vi "sequential on_off - v2.vi"() -> ()   [LabVIEW 2018]
doc: "Manually blink and LED attached to a digital output channel of a LINX device by clicking and LED control in LabVIEW."
uses:
  <vilib>/MakerHub/LINX/Public/Peripherals/Digital/Digital Write 1 Chan.vi
  <vilib>/MakerHub/LINX/Public/Peripherals/Digital/Digital Write N Chans.vi
  <vilib>/MakerHub/LINX/Private/Local IO/LinxDigitalWrite.vi
  <vilib>/MakerHub/LINX/Public/Utilities/Check Channel.vi
  <vilib>/MakerHub/LINX/Public/Utilities/Open Serial.vi
  <vilib>/MakerHub/LINX/Private/Utilties/Generate Error.vi
  <vilib>/MakerHub/LINX/LMH-LINX.lvlib
panel:
  in  "Chnl_1":bool
  in  "Chnl_2":bool
  in  "Chnl_4":bool
  in  "Chnl_3":bool
  in  "Delay (ms)":dbl
  in  "Mode Selection":enum32{"Manual Control", "Sequential Control"}(radio)
  out "ch_4":bool
  out "ch_3":bool
  out "ch_2":bool
  out "ch_1":bool
  in  "Reset valves":bool
  out "id_8":bool
  out "id_7":bool
  out "id_6":bool
  out "id_5":bool
  out "id_4":bool
  out "id_3":bool
  out "id_2":bool
  out "id_1":bool
  in  "stop":bool
  in  "Valve 8":bool
  in  "Valve 7":bool
  in  "Valve 6":bool
  in  "Valve 5":bool
  in  "Valve 4":bool
  in  "Valve 3":bool
  in  "Valve 2":bool
  in  "Valve_1":bool
  in  "Serial Port":refnum<visa-resource-name>
  # "Manual Control:"
  # "LINX Device Settings"
  # "Sequential Control:"
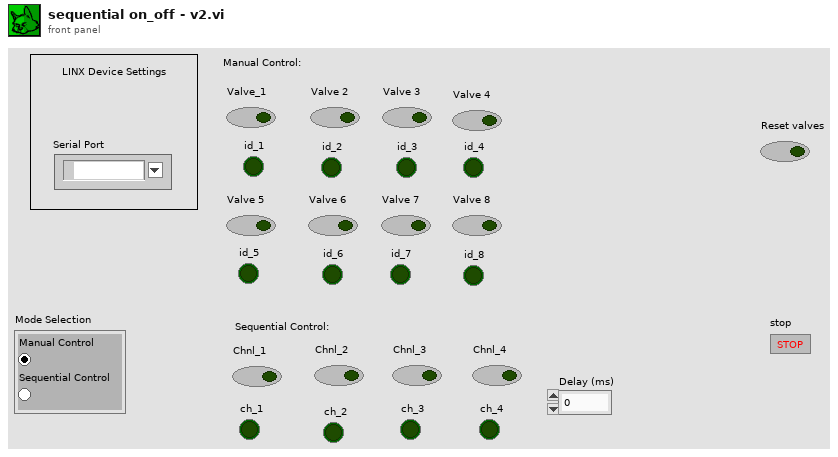
[diagram p1: front panel]
types:
  T1 = typedef "LMH-LINX.lvlib/LINX Ref.ctl" = cluster{"IO":T2, "Interface":T3, "LINX Device Config":T4}
  T2 = typedef "LMH-LINX.lvlib/Platform.ctl" = enum16{"Remote", "Local"}
  T3 = typedef "LMH-LINX.lvlib/Interface.ctl" = enum16{"Serial", "TCP"}
  T4 = typedef "LMH-LINX.lvlib/Device.lvlib/LINX Device Config.ctl" = cluster{"Interface":T3, "COM Port":refnum<visa-resource-name>, "TCP Configuration":T5, "Device Family":u8, "Device ID":u8, "Device Name":string, "TCP Ref":refnum<k5>, "Channels":T6}
  T5 = typedef "LMH-LINX.lvlib/Device.lvlib/TCP Config.ctl" = cluster{"IP Address":string, "Port":u16}
  T6 = typedef "LMH-LINX.lvlib/Channels.ctl" = cluster{"DI":u8[], "DO":u8[], "AI":u8[], "AO":u8[], "PWM":u8[], "QE":u8[], "UART":u8[], "I2C 2":u8[], "SPI":u8[], "CAN":u8[], "Servo":u8[], "AI Ref (V)":dbl, "AI Resolution (Bits)":u8, "AO Ref (V)":dbl, "AO Resolution (Bits)":u8}
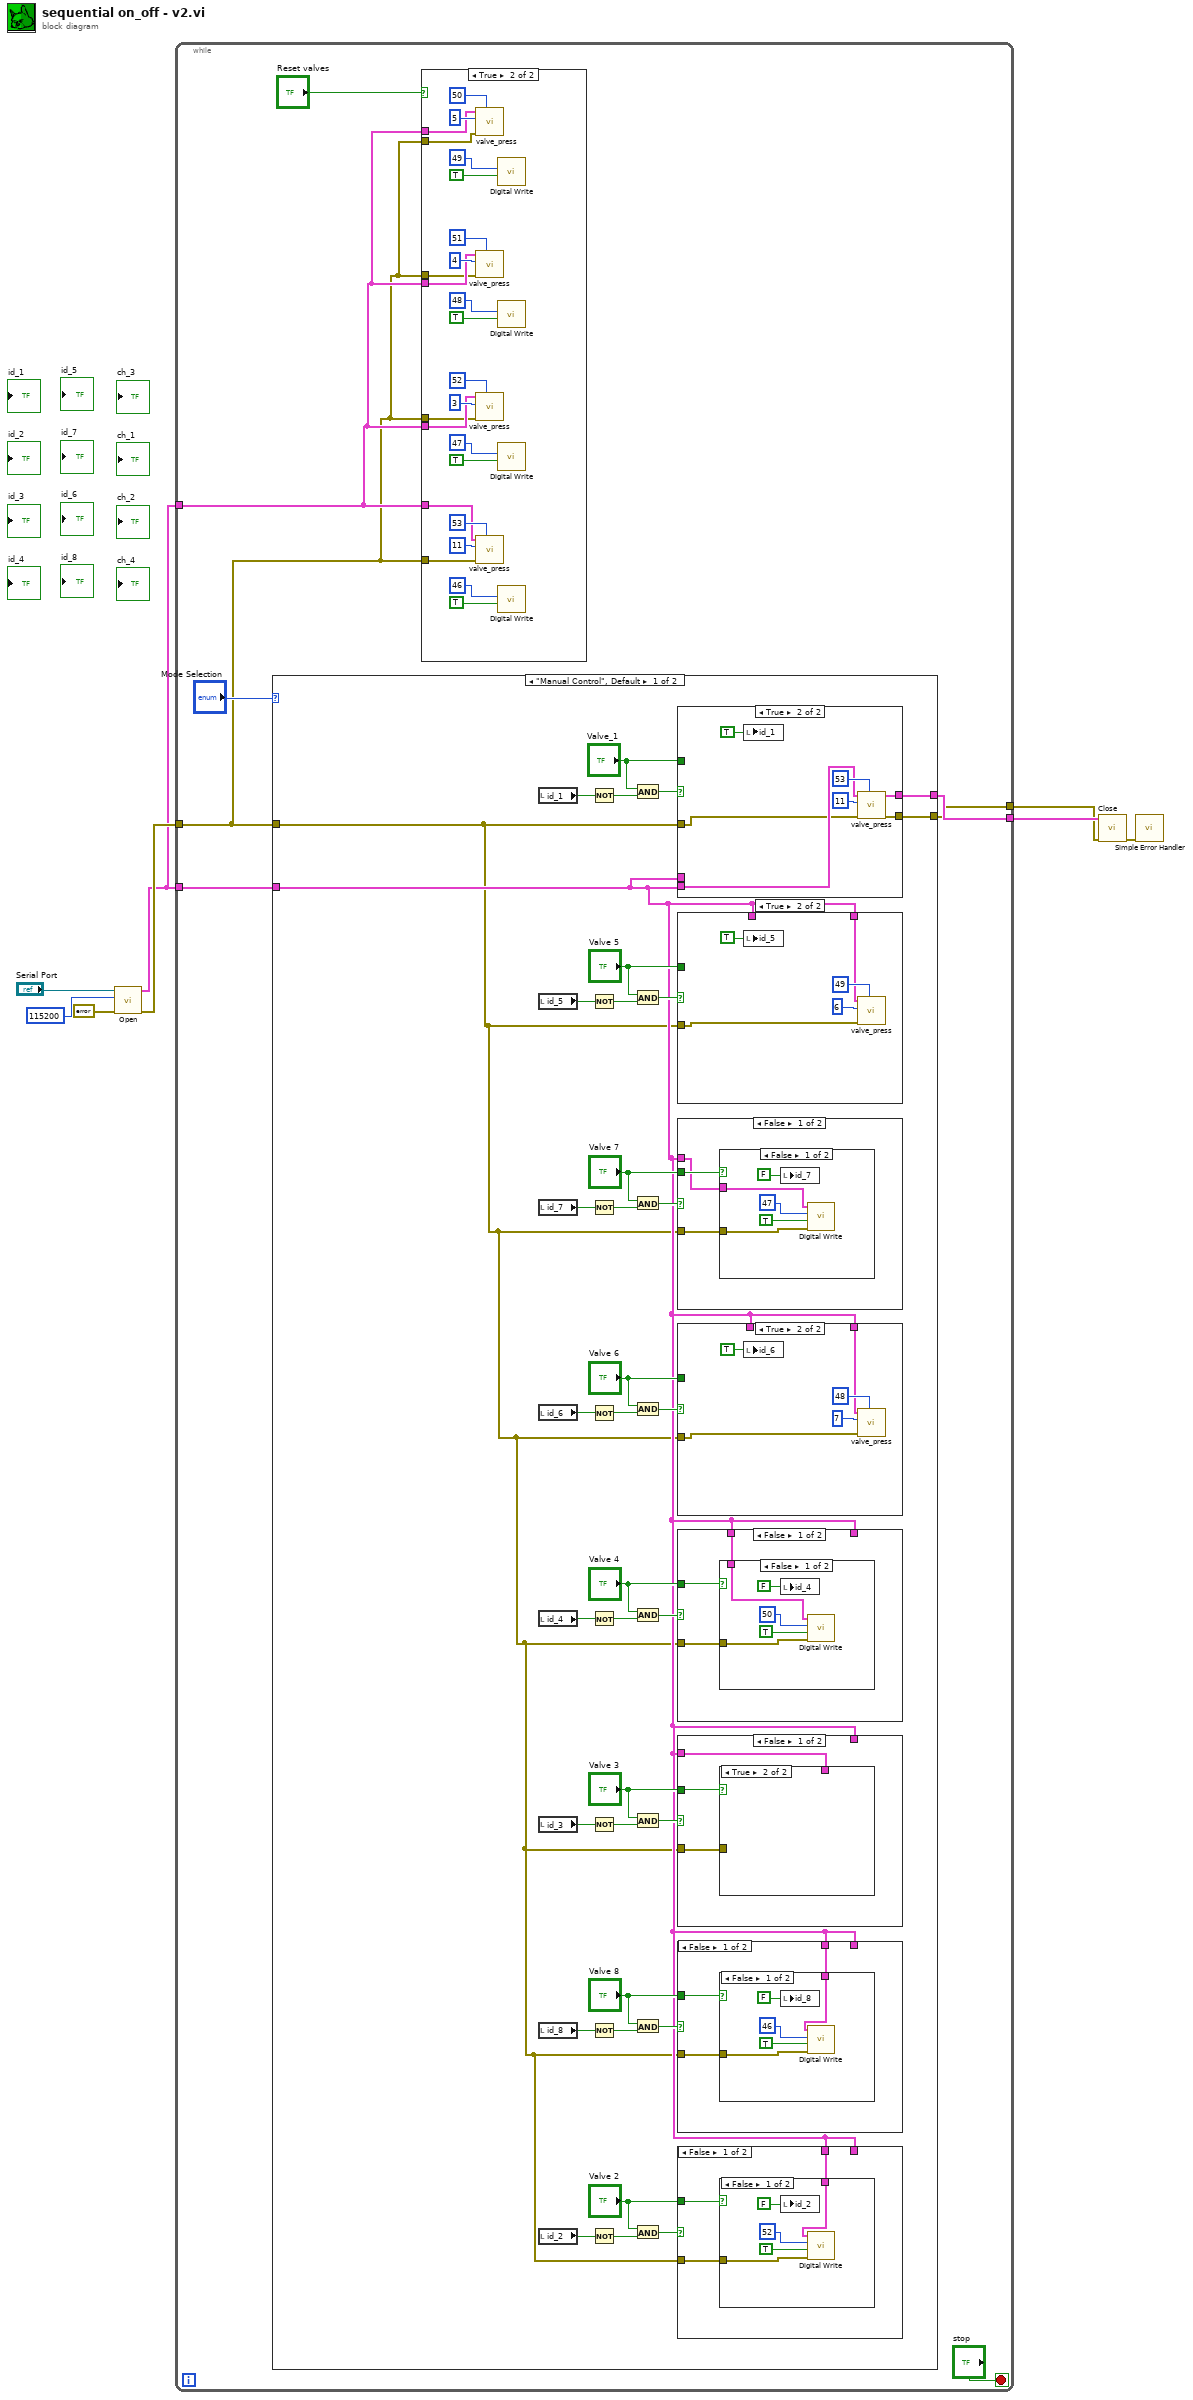
[diagram p0: block diagram]
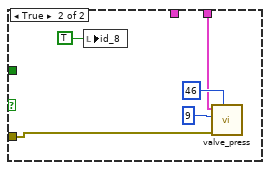
[diagram p3: hidden frame]
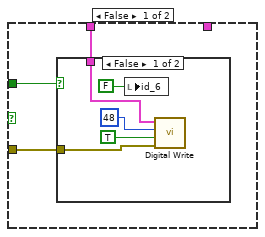
[diagram p4: hidden frame]
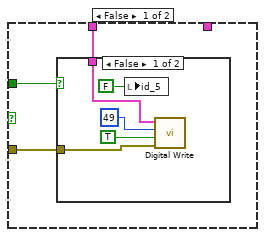
[diagram p6: hidden frame]
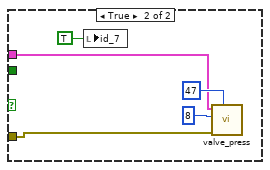
[diagram p9: hidden frame]
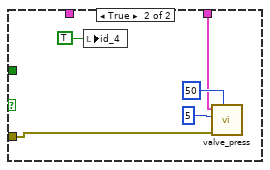
[diagram p11: hidden frame]
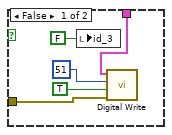
[diagram p12: hidden frame]
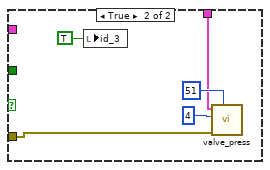
[diagram p13: hidden frame]
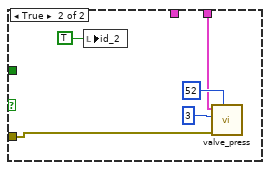
[diagram p15: hidden frame]
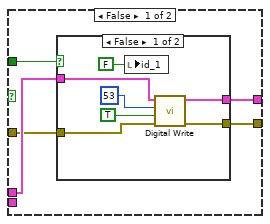
[diagram p16: hidden frame]
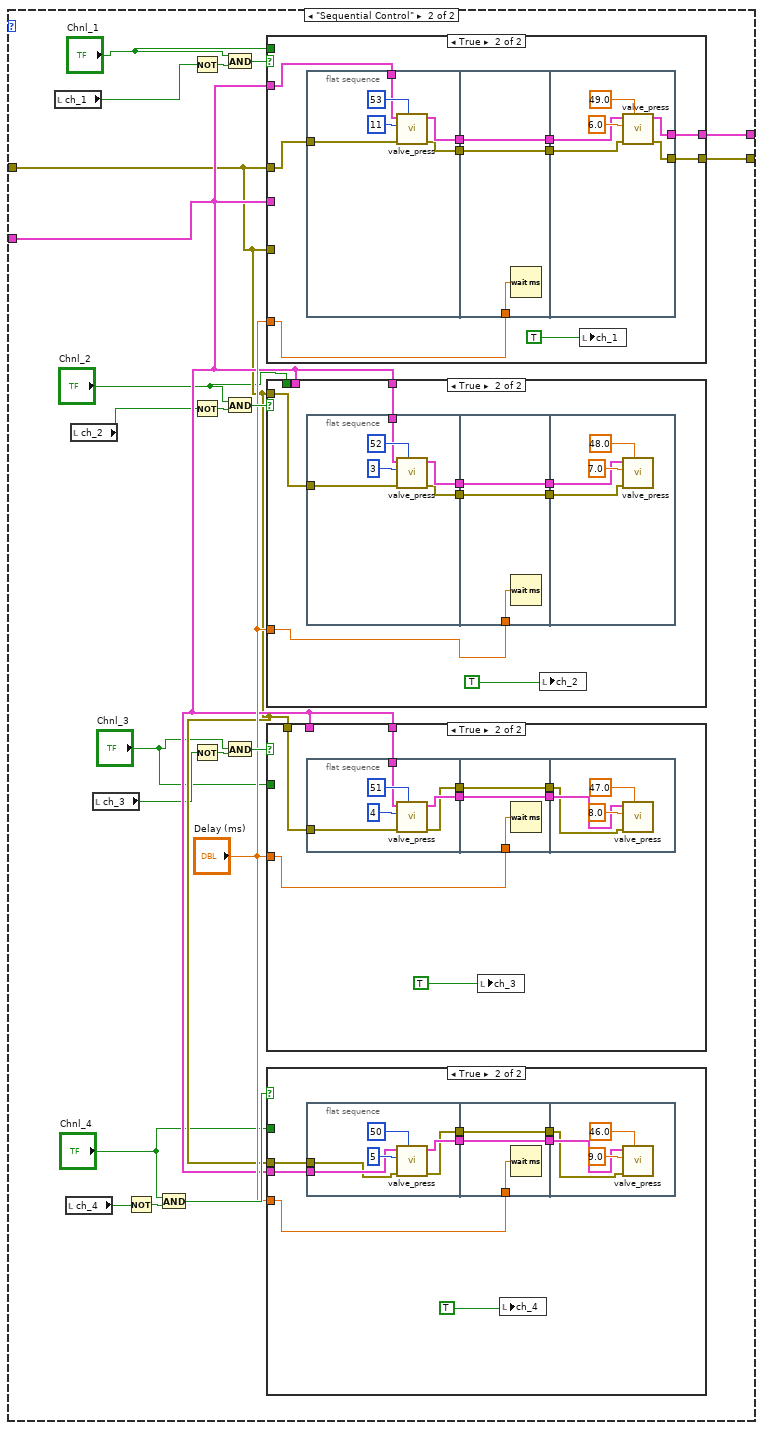
[diagram p18: hidden frame]
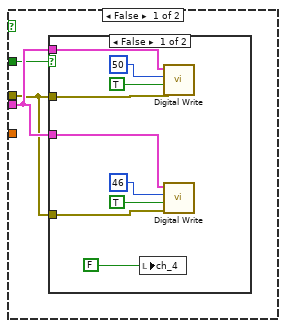
[diagram p19: hidden frame]
diagram:
  n1 = call-poly <vilib>:"Open.vi"("Error In"=errorcluster {"status"=FALSE, "code"=0, "source"=""}, "Baud Rate Override"=u32 115200, "Serial Port"="Serial Port") -> ("Error Out"=w4:errorcluster, "LINX Resource"=w1:T1)  [unwired: 6 in, 1 out]
  n2 = while {
    tunnel: w1 -> [w13]
    tunnel: w4 -> [w9]
    tunnel: [w12] -> w3
    tunnel: [w11] -> w2
    tunnel: w1 -> [w10]
    stop <- "stop" stop-if-true
    n3 = case shown="\"Manual Control\", Default" "Mode Selection" {
      tunnel: [w20 w176] -> w12
      tunnel: [w19 w175] -> w11
      tunnel: w13 -> [w18 w174]
      tunnel: w9 -> [w17 w173]
      frame "Manual Control", Default {
        n4 = local read "id_1"() -> (w22:bool)
        n5 = local read "id_5"() -> (w35:bool)
        n6 = local read "id_7"() -> (w37:bool)
        n7 = local read "id_6"() -> (w36:bool)
        n8 = local read "id_4"() -> (w34:bool)
        n9 = local read "id_3"() -> (w33:bool)
        n10 = local read "id_8"() -> (w38:bool)
        n11 = local read "id_2"() -> (w26:bool)
        n12 = Not(x=w22) -> (.not. x?=w23:bool)
        n13 = Not(x=w35) -> (.not. x?=w45:bool)
        n14 = Not(x=w37) -> (.not. x?=w41:bool)
        n15 = Not(x=w36) -> (.not. x?=w43:bool)
        n16 = Not(x=w34) -> (.not. x?=w31:bool)
        n17 = Not(x=w33) -> (.not. x?=w28:bool)
        n18 = Not(x=w38) -> (.not. x?=w39:bool)
        n19 = Not(x=w26) -> (.not. x?=w25:bool)
        n20 = And(x="Valve_1", y=w23) -> (x .and. y?=w21:bool)
        n21 = And(x="Valve 5", y=w45) -> (x .and. y?=w46:bool)
        n22 = And(x="Valve 7", y=w41) -> (x .and. y?=w42:bool)
        n23 = And(x="Valve 6", y=w43) -> (x .and. y?=w44:bool)
        n24 = And(x="Valve 4", y=w31) -> (x .and. y?=w32:bool)
        n25 = And(x="Valve 3", y=w28) -> (x .and. y?=w29:bool)
        n26 = And(x="Valve 8", y=w39) -> (x .and. y?=w40:bool)
        n27 = And(x="Valve 2", y=w25) -> (x .and. y?=w24:bool)
        n28 = case shown="True" w21 {
          tunnel: [w147 w164] -> w20
          tunnel: [w148 w163] -> w19
          tunnel: "Valve_1" -> [w146 _]
          tunnel: w18 -> [_ w159]
          tunnel: w18 -> [w145 _]
          tunnel: w17 -> [w144 w158]
          frame False {
            n29 = case shown="False" w146 {
              tunnel: [w152 w156] -> w148
              tunnel: [w151 w157] -> w147
              tunnel: w145 -> [w150 w157]
              tunnel: w144 -> [w149 w156]
              frame False {
                n30 = local write "id_1"(FALSE) -> ()
                n31 = call-poly <vilib>:"Digital Write.vi"("Error In"=w149, "Output Value"=TRUE, "DO Channel"=u8 53, "LINX Resource"=w150) -> ("Error Out"=w152:errorcluster, "LINX Resource"=w151:T1)  [unwired: 6 in]
              }
              frame True {
              }
            }
          }
          frame True {
            n32 = local write "id_1"(TRUE) -> ()
            n33 = call "valve_press.vi"("power"=53, "error in (no error)"=w158, "trigger"=11, "LINX Resource in"=w159) -> ("error out"=w163:errorcluster, "LINX Resource out"=w164:T1)  [unwired: 6 in]
          }
        }
        n34 = case shown="True" w46 {
          tunnel: "Valve 5" -> [w81 _]
          tunnel: w18 -> [_ w88]
          tunnel: w18 -> [w80 _]
          tunnel: w17 -> [w79 w87]
          frame False {
            n35 = case shown="False" w81 {
              tunnel: w80 -> [w83 _]
              tunnel: w79 -> [w82 _]
              frame False {
                n36 = local write "id_5"(FALSE) -> ()
                n37 = call-poly <vilib>:"Digital Write.vi"("Error In"=w82, "Output Value"=TRUE, "DO Channel"=u8 49, "LINX Resource"=w83) -> ()  [unwired: 6 in, 2 out]
              }
              frame True {
              }
            }
          }
          frame True {
            n38 = local write "id_5"(TRUE) -> ()
            n39 = call "valve_press.vi"("power"=49, "error in (no error)"=w87, "trigger"=6, "LINX Resource in"=w88) -> ()  [unwired: 6 in, 2 out]
          }
        }
        n40 = case shown="False" w42 {
          tunnel: "Valve 7" -> [w94 _]
          tunnel: w18 -> [w93 w101]
          tunnel: w17 -> [w92 w100]
          frame False {
            n41 = case shown="False" w94 {
              tunnel: w93 -> [w96 _]
              tunnel: w92 -> [w95 _]
              frame False {
                n42 = local write "id_7"(FALSE) -> ()
                n43 = call-poly <vilib>:"Digital Write.vi"("Error In"=w95, "Output Value"=TRUE, "DO Channel"=u8 47, "LINX Resource"=w96) -> ()  [unwired: 6 in, 2 out]
              }
              frame True {
              }
            }
          }
          frame True {
            n44 = local write "id_7"(TRUE) -> ()
            n45 = call "valve_press.vi"("power"=47, "error in (no error)"=w100, "trigger"=8, "LINX Resource in"=w101) -> ()  [unwired: 6 in, 2 out]
          }
        }
        n46 = case shown="True" w44 {
          tunnel: "Valve 6" -> [w68 _]
          tunnel: w18 -> [_ w75]
          tunnel: w18 -> [w67 _]
          tunnel: w17 -> [w66 w74]
          frame False {
            n47 = case shown="False" w68 {
              tunnel: w67 -> [w70 _]
              tunnel: w66 -> [w69 _]
              frame False {
                n48 = local write "id_6"(FALSE) -> ()
                n49 = call-poly <vilib>:"Digital Write.vi"("Error In"=w69, "Output Value"=TRUE, "DO Channel"=u8 48, "LINX Resource"=w70) -> ()  [unwired: 6 in, 2 out]
              }
              frame True {
              }
            }
          }
          frame True {
            n50 = local write "id_6"(TRUE) -> ()
            n51 = call "valve_press.vi"("power"=48, "error in (no error)"=w74, "trigger"=7, "LINX Resource in"=w75) -> ()  [unwired: 6 in, 2 out]
          }
        }
        n52 = case shown="False" w32 {
          tunnel: "Valve 4" -> [w107 _]
          tunnel: w18 -> [_ w114]
          tunnel: w18 -> [w106 _]
          tunnel: w17 -> [w105 w113]
          frame False {
            n53 = case shown="False" w107 {
              tunnel: w106 -> [w109 _]
              tunnel: w105 -> [w108 _]
              frame False {
                n54 = local write "id_4"(FALSE) -> ()
                n55 = call-poly <vilib>:"Digital Write.vi"("Error In"=w108, "Output Value"=TRUE, "DO Channel"=u8 50, "LINX Resource"=w109) -> ()  [unwired: 6 in, 2 out]
              }
              frame True {
              }
            }
          }
          frame True {
            n56 = local write "id_4"(TRUE) -> ()
            n57 = call "valve_press.vi"("power"=50, "error in (no error)"=w113, "trigger"=5, "LINX Resource in"=w114) -> ()  [unwired: 6 in, 2 out]
          }
        }
        n58 = case shown="False" w29 {
          tunnel: "Valve 3" -> [w120 _]
          tunnel: w18 -> [_ w127]
          tunnel: w18 -> [w119 _]
          tunnel: w17 -> [w118 w126]
          frame False {
            n59 = case shown="True" w120 {
              tunnel: w119 -> [w122 _]
              tunnel: w118 -> [w121 _]
              frame False {
                n60 = local write "id_3"(FALSE) -> ()
                n61 = call-poly <vilib>:"Digital Write.vi"("Error In"=w121, "Output Value"=TRUE, "DO Channel"=u8 51, "LINX Resource"=w122) -> ()  [unwired: 6 in, 2 out]
              }
              frame True {
              }
            }
          }
          frame True {
            n62 = local write "id_3"(TRUE) -> ()
            n63 = call "valve_press.vi"("power"=51, "error in (no error)"=w126, "trigger"=4, "LINX Resource in"=w127) -> ()  [unwired: 6 in, 2 out]
          }
        }
        n64 = case shown="False" w40 {
          tunnel: "Valve 8" -> [w55 _]
          tunnel: w18 -> [_ w62]
          tunnel: w18 -> [w54 _]
          tunnel: w17 -> [w53 w61]
          frame False {
            n65 = case shown="False" w55 {
              tunnel: w54 -> [w57 _]
              tunnel: w53 -> [w56 _]
              frame False {
                n66 = local write "id_8"(FALSE) -> ()
                n67 = call-poly <vilib>:"Digital Write.vi"("Error In"=w56, "Output Value"=TRUE, "DO Channel"=u8 46, "LINX Resource"=w57) -> ()  [unwired: 6 in, 2 out]
              }
              frame True {
              }
            }
          }
          frame True {
            n68 = local write "id_8"(TRUE) -> ()
            n69 = call "valve_press.vi"("power"=46, "error in (no error)"=w61, "trigger"=9, "LINX Resource in"=w62) -> ()  [unwired: 6 in, 2 out]
          }
        }
        n70 = case shown="False" w24 {
          tunnel: "Valve 2" -> [w133 _]
          tunnel: w18 -> [_ w140]
          tunnel: w18 -> [w132 _]
          tunnel: w17 -> [w131 w139]
          frame False {
            n71 = case shown="False" w133 {
              tunnel: w132 -> [w135 _]
              tunnel: w131 -> [w134 _]
              frame False {
                n72 = local write "id_2"(FALSE) -> ()
                n73 = call-poly <vilib>:"Digital Write.vi"("Error In"=w134, "Output Value"=TRUE, "DO Channel"=u8 52, "LINX Resource"=w135) -> ()  [unwired: 6 in, 2 out]
              }
              frame True {
              }
            }
          }
          frame True {
            n74 = local write "id_2"(TRUE) -> ()
            n75 = call "valve_press.vi"("power"=52, "error in (no error)"=w139, "trigger"=3, "LINX Resource in"=w140) -> ()  [unwired: 6 in, 2 out]
          }
        }
      }
      frame "Sequential Control" {
        n76 = local read "ch_1"() -> (w172:bool)
        n77 = local read "ch_4"() -> (w166:bool)
        n78 = local read "ch_2"() -> (w169:bool)
        n79 = local read "ch_3"() -> (w168:bool)
        n80 = Not(x=w166) -> (.not. x?=w179:bool)
        n81 = And(x="Chnl_4", y=w179) -> (x .and. y?=w178:bool)
        n82 = Not(x=w172) -> (.not. x?=w185:bool)
        n83 = Not(x=w169) -> (.not. x?=w183:bool)
        n84 = Not(x=w168) -> (.not. x?=w181:bool)
        n85 = And(x="Chnl_1", y=w185) -> (x .and. y?=w184:bool)
        n86 = And(x="Chnl_2", y=w183) -> (x .and. y?=w182:bool)
        n87 = And(x="Chnl_3", y=w181) -> (x .and. y?=w180:bool)
        n88 = case shown="True" w184 {
          tunnel: "Delay (ms)" -> [_ w314]
          tunnel: w174 -> [w291 w313]
          tunnel: w173 -> [w290 w312]
          tunnel: w174 -> [w289 _]
          tunnel: w173 -> [w288 _]
          tunnel: [w287 w307] -> w176
          tunnel: [w286 w306] -> w175
          tunnel: "Chnl_1" -> [w285 _]
          frame False {
            n89 = case shown="False" w285 {
              tunnel: w291 -> [w298 w304]
              tunnel: w290 -> [w297 w303]
              tunnel: w289 -> [w296 _]
              tunnel: w288 -> [w295 _]
              tunnel: [w294 w304] -> w287
              tunnel: [w293 w303] -> w286
              frame False {
                n90 = local write "ch_1"(FALSE) -> ()
                n91 = call-poly <vilib>:"Digital Write.vi"("Error In"=w297, "Output Value"=TRUE, "DO Channel"=u8 53, "LINX Resource"=w298) -> ("Error Out"=w293:errorcluster, "LINX Resource"=w294:T1)  [unwired: 6 in]
                n92 = call-poly <vilib>:"Digital Write.vi"("Error In"=w295, "Output Value"=TRUE, "DO Channel"=u8 49, "LINX Resource"=w296) -> ()  [unwired: 6 in, 2 out]
              }
              frame True {
              }
            }
          }
          frame True {
            n93 = flat-sequence {
              tunnel: w313 -> [w318]
              tunnel: w312 -> [w317]
              tunnel: [w316] -> w310
              tunnel: [w315] -> w308
              tunnel: w314 -> [w323]
              tunnel: [w322] -> w311
              tunnel: w310 -> [w322]
              tunnel: [w321] -> w309
              tunnel: w308 -> [w321]
              tunnel: w311 -> [w327]
              tunnel: w309 -> [w326]
              tunnel: [w325] -> w307
              tunnel: [w324] -> w306
              frame #0 {
                n94 = call "valve_press.vi"("power"=53, "error in (no error)"=w317, "trigger"=11, "LINX Resource in"=w318) -> ("error out"=w315:errorcluster, "LINX Resource out"=w316:T1)  [unwired: 6 in]
              }
              frame #1 {
                n95 = Wait (ms)(milliseconds to wait=w323) -> ()  [unwired: 1 out]
              }
              frame #2 {
                n96 = call "valve_press.vi"("power"=49.0, "error in (no error)"=w326, "trigger"=6.0, "LINX Resource in"=w327) -> ("error out"=w324:errorcluster, "LINX Resource out"=w325:T1)  [unwired: 6 in]
              }
            }
            n97 = local write "ch_1"(TRUE) -> ()
          }
        }
        n98 = case shown="True" w182 {
          tunnel: "Delay (ms)" -> [_ w271]
          tunnel: w174 -> [w255 w270]
          tunnel: w173 -> [w253 w269]
          tunnel: w174 -> [w254 _]
          tunnel: "Chnl_2" -> [w252 _]
          frame False {
            n99 = case shown="False" w252 {
              tunnel: w255 -> [w259 _]
              tunnel: w254 -> [w258 _]
              tunnel: w253 -> [w257 _]
              frame False {
                n100 = local write "ch_2"(FALSE) -> ()
                n101 = call-poly <vilib>:"Digital Write.vi"("Error In"=w257, "Output Value"=TRUE, "DO Channel"=u8 48, "LINX Resource"=w259) -> ()  [unwired: 6 in, 2 out]
                n102 = call-poly <vilib>:"Digital Write.vi"("Error In"=w257, "Output Value"=TRUE, "DO Channel"=u8 52, "LINX Resource"=w258) -> ()  [unwired: 6 in, 2 out]
              }
              frame True {
              }
            }
          }
          frame True {
            n103 = flat-sequence {
              tunnel: w270 -> [w275]
              tunnel: w269 -> [w274]
              tunnel: [w273] -> w267
              tunnel: [w272] -> w265
              tunnel: w271 -> [w280]
              tunnel: [w279] -> w268
              tunnel: w267 -> [w279]
              tunnel: [w278] -> w266
              tunnel: w265 -> [w278]
              tunnel: w268 -> [w282]
              tunnel: w266 -> [w281]
              frame #0 {
                n104 = call "valve_press.vi"("power"=52, "error in (no error)"=w274, "trigger"=3, "LINX Resource in"=w275) -> ("error out"=w272:errorcluster, "LINX Resource out"=w273:T1)  [unwired: 6 in]
              }
              frame #1 {
                n105 = Wait (ms)(milliseconds to wait=w280) -> ()  [unwired: 1 out]
              }
              frame #2 {
                n106 = call "valve_press.vi"("power"=48.0, "error in (no error)"=w281, "trigger"=7.0, "LINX Resource in"=w282) -> ()  [unwired: 6 in, 2 out]
              }
            }
            n107 = local write "ch_2"(TRUE) -> ()
          }
        }
        n108 = case shown="True" w180 {
          tunnel: "Delay (ms)" -> [_ w238]
          tunnel: w174 -> [w222 w237]
          tunnel: w173 -> [w220 w234]
          tunnel: w174 -> [w221 _]
          tunnel: "Chnl_3" -> [w219 _]
          frame False {
            n109 = case shown="False" w219 {
              tunnel: w222 -> [w226 _]
              tunnel: w221 -> [w225 _]
              tunnel: w220 -> [w224 _]
              frame False {
                n110 = call-poly <vilib>:"Digital Write.vi"("Error In"=w224, "Output Value"=TRUE, "DO Channel"=u8 51, "LINX Resource"=w226) -> ()  [unwired: 6 in, 2 out]
                n111 = call-poly <vilib>:"Digital Write.vi"("Error In"=w224, "Output Value"=TRUE, "DO Channel"=u8 47, "LINX Resource"=w225) -> ()  [unwired: 6 in, 2 out]
                n112 = local write "ch_3"(FALSE) -> ()
              }
              frame True {
              }
            }
          }
          frame True {
            n113 = flat-sequence {
              tunnel: w237 -> [w242]
              tunnel: [w241] -> w235
              tunnel: w234 -> [w240]
              tunnel: [w239] -> w232
              tunnel: w238 -> [w247]
              tunnel: [w246] -> w236
              tunnel: w235 -> [w246]
              tunnel: [w245] -> w233
              tunnel: w232 -> [w245]
              tunnel: w236 -> [w249]
              tunnel: w233 -> [w248]
              frame #0 {
                n114 = call "valve_press.vi"("power"=51, "error in (no error)"=w240, "trigger"=4, "LINX Resource in"=w242) -> ("error out"=w239:errorcluster, "LINX Resource out"=w241:T1)  [unwired: 6 in]
              }
              frame #1 {
                n115 = Wait (ms)(milliseconds to wait=w247) -> ()  [unwired: 1 out]
              }
              frame #2 {
                n116 = call "valve_press.vi"("power"=47.0, "error in (no error)"=w248, "trigger"=8.0, "LINX Resource in"=w249) -> ()  [unwired: 6 in, 2 out]
              }
            }
            n117 = local write "ch_3"(TRUE) -> ()
          }
        }
        n118 = case shown="True" w178 {
          tunnel: "Delay (ms)" -> [_ w205]
          tunnel: w174 -> [w188 w204]
          tunnel: w173 -> [w187 w203]
          tunnel: "Chnl_4" -> [w186 _]
          frame False {
            n119 = case shown="False" w186 {
              tunnel: w188 -> [w193 _]
              tunnel: w187 -> [w192 _]
              tunnel: w188 -> [w191 _]
              tunnel: w187 -> [w190 _]
              frame False {
                n120 = local write "ch_4"(FALSE) -> ()
                n121 = call-poly <vilib>:"Digital Write.vi"("Error In"=w192, "Output Value"=TRUE, "DO Channel"=u8 50, "LINX Resource"=w193) -> ()  [unwired: 6 in, 2 out]
                n122 = call-poly <vilib>:"Digital Write.vi"("Error In"=w190, "Output Value"=TRUE, "DO Channel"=u8 46, "LINX Resource"=w191) -> ()  [unwired: 6 in, 2 out]
              }
              frame True {
              }
            }
          }
          frame True {
            n123 = flat-sequence {
              tunnel: w204 -> [w209]
              tunnel: w203 -> [w208]
              tunnel: [w207] -> w201
              tunnel: [w206] -> w199
              tunnel: w205 -> [w214]
              tunnel: [w213] -> w202
              tunnel: w201 -> [w213]
              tunnel: [w212] -> w200
              tunnel: w199 -> [w212]
              tunnel: w202 -> [w216]
              tunnel: w200 -> [w215]
              frame #0 {
                n124 = call "valve_press.vi"("power"=50, "error in (no error)"=w208, "trigger"=5, "LINX Resource in"=w209) -> ("error out"=w206:errorcluster, "LINX Resource out"=w207:T1)  [unwired: 6 in]
              }
              frame #1 {
                n125 = Wait (ms)(milliseconds to wait=w214) -> ()  [unwired: 1 out]
              }
              frame #2 {
                n126 = call "valve_press.vi"("power"=46.0, "error in (no error)"=w215, "trigger"=9.0, "LINX Resource in"=w216) -> ()  [unwired: 6 in, 2 out]
              }
            }
            n127 = local write "ch_4"(TRUE) -> ()
          }
        }
      }
    }
    n128 = case shown="True" "Reset valves" {
      tunnel: w10 -> [_ w337]
      tunnel: w9 -> [_ w336]
      tunnel: w10 -> [_ w335]
      tunnel: w9 -> [_ w334]
      tunnel: w10 -> [_ w333]
      tunnel: w9 -> [_ w332]
      tunnel: w10 -> [_ w331]
      tunnel: w9 -> [_ w330]
      frame False {
      }
      frame True {
        n129 = call "valve_press.vi"("power"=50, "error in (no error)"=w330, "trigger"=5, "LINX Resource in"=w331) -> ()  [unwired: 6 in, 2 out]
        n130 = call "valve_press.vi"("power"=51, "error in (no error)"=w332, "trigger"=4, "LINX Resource in"=w333) -> ()  [unwired: 6 in, 2 out]
        n131 = call "valve_press.vi"("power"=52, "error in (no error)"=w334, "trigger"=3, "LINX Resource in"=w335) -> ()  [unwired: 6 in, 2 out]
        n132 = call "valve_press.vi"("power"=53, "error in (no error)"=w336, "trigger"=11, "LINX Resource in"=w337) -> ()  [unwired: 6 in, 2 out]
        n133 = call-poly <vilib>:"Digital Write.vi"("Output Value"=TRUE, "DO Channel"=u8 49) -> ()  [unwired: 8 in, 2 out]
        n134 = call-poly <vilib>:"Digital Write.vi"("Output Value"=TRUE, "DO Channel"=u8 48) -> ()  [unwired: 8 in, 2 out]
        n135 = call-poly <vilib>:"Digital Write.vi"("Output Value"=TRUE, "DO Channel"=u8 47) -> ()  [unwired: 8 in, 2 out]
        n136 = call-poly <vilib>:"Digital Write.vi"("Output Value"=TRUE, "DO Channel"=u8 46) -> ()  [unwired: 8 in, 2 out]
      }
    }
  }
  n137 = call <vilib>:"Close.vi"("Error In"=w2, "LINX Resource"=w3) -> ("Error Out"=w7:errorcluster)  [unwired: 9 in]
  n138 = call <vilib>:"Simple Error Handler.vi"("error in (no error)"=w7) -> ()  [unwired: 4 in, 5 out]
